vi "Lin Daten verwalten.vi"(6 "Aktionen":T6, 7 "Dateiname":string, 8 "Pfad":string, 9 "Stufen Tabelle":T5, 10 "Punkte umkehren":bool, 11 "Lin Daten":T1 {"CalGas Eingang" items=["Cal Gas 1", "Cal Gas 2", "Cal Gas 3"]; "Max Fehler (Sollwert)" format="%#_5g"; "Zeitdauer Stufe" format="%#_5g"; "Anzahl Stufen" format="%#_5g"; "Verdünnungsgas" items=["N2", "O2"]}) -> (0 "Pfad":string, 1 "Stufen Tabelle":T5, 2 "Lin Daten einzeln":T1 {"CalGas Eingang" items=["Cal Gas 1", "Cal Gas 2", "Cal Gas 3"]; "Max Fehler (Sollwert)" format="%#_5g"; "Zeitdauer Stufe" format="%#_5g"; "Anzahl Stufen" format="%#_5g"; "Verdünnungsgas" items=["N2", "O2"]}, 3 "Gefunden?":bool, 4 "Punkte umkehren":bool, 5 "Dateiname":string)   [LabVIEW 2020, in "Linearisierung v2.lvlib" / "Gasteiler.lvlib"]
uses:
  Gasteiler.lvlib
  Lin Daten verwalten Aktionen.ctl
  Lin Daten.ctl
  Visualisierungs Elemente/String - Eingabefeld.ctl
  Visualisierungs Elemente/Zahlen-Eingabefeld.ctl
  Stufen Tabelle.ctl
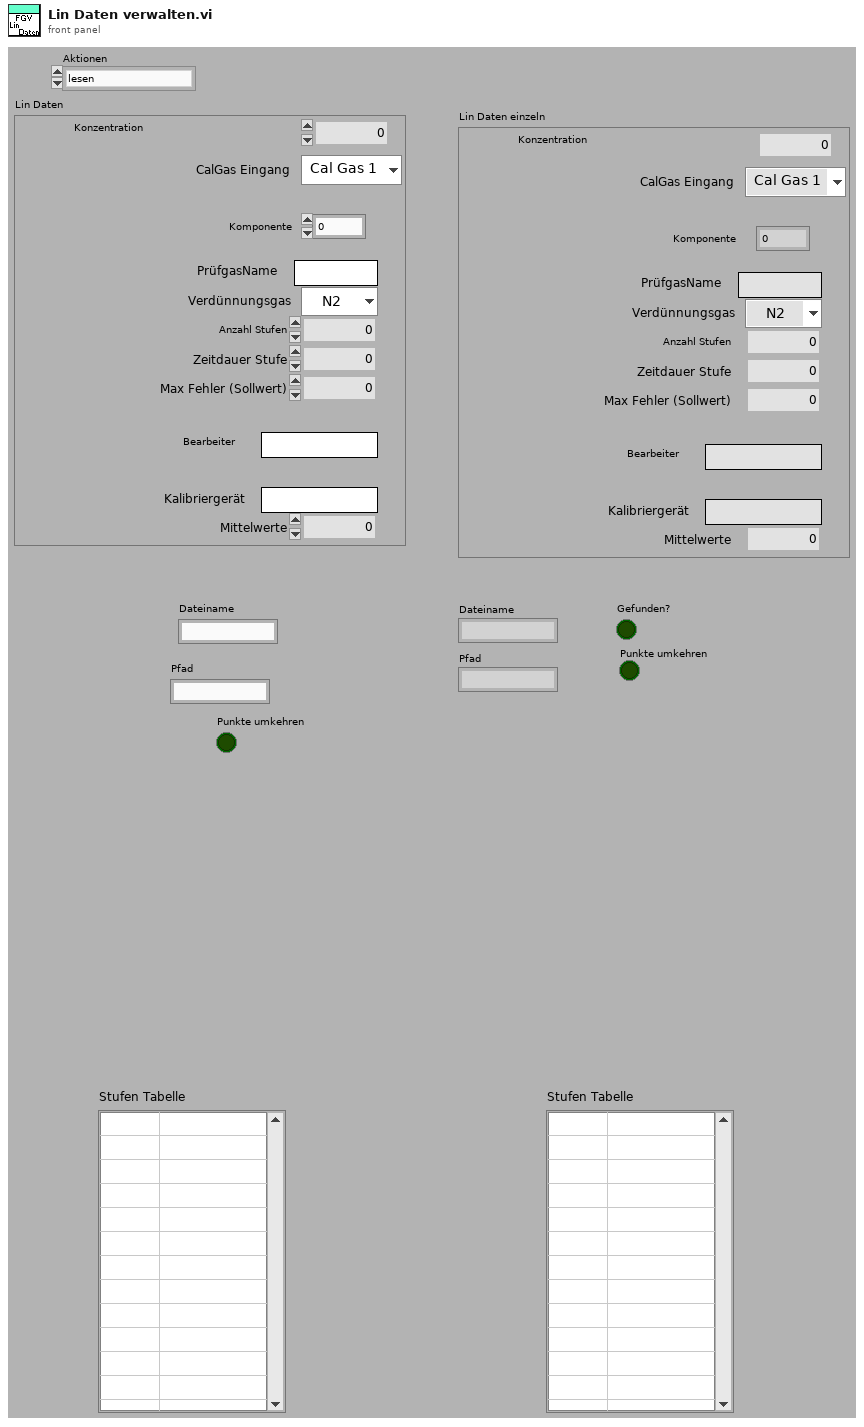
[diagram p1: front panel]
types:
  T1 = typedef "Linearisierung v2.lvlib/Gasteiler.lvlib/Lin Daten.ctl" = cluster{"PrüfgasName":T2, "Verdünnungsgas":T3, "Anzahl Stufen":T4, "Zeitdauer Stufe":T4, "Max Fehler (Sollwert)":T4, "Bearbeiter":T2, "Kalibriergerät":T2, "Mittelwerte":i32, "Komponente":u16, "CalGas Eingang":u16, "Konzentration":sgl}
  T2 = typedef "String - Eingabefeld.ctl" = string
  T3 = typedef "Linearisierung v2.lvlib/Gasteiler.lvlib/Prüfgas in.ctl" = u16
  T4 = typedef "Zahlen-Eingabefeld.ctl" = sgl
  T5 = typedef "Linearisierung v2.lvlib/Gasteiler.lvlib/Stufen Tabelle.ctl" = string[][]
  T6 = typedef "Linearisierung v2.lvlib/Gasteiler.lvlib/Lin Daten verwalten Aktionen.ctl" = enum16{"lesen", "speichern", "laden", "Lin Daten schr.", "Stufen Tabelle", "Lin Name AK", "Lin Pfad AK", "Umkehren"}
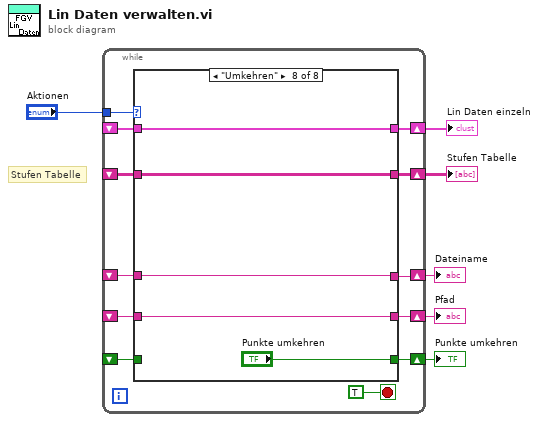
[diagram p0: block diagram]
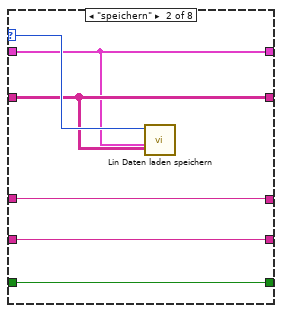
[diagram p3: hidden frame]
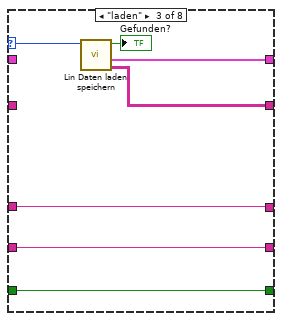
[diagram p4: hidden frame]
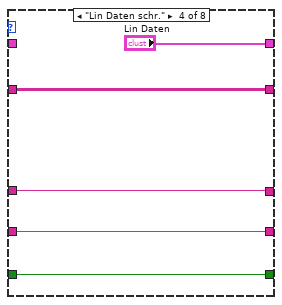
[diagram p5: hidden frame]
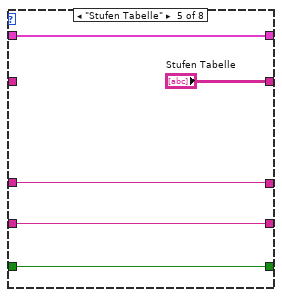
[diagram p6: hidden frame]
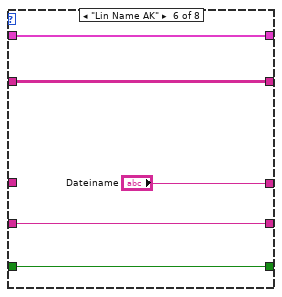
[diagram p7: hidden frame]
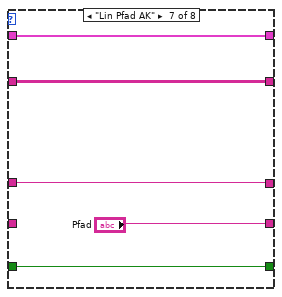
[diagram p8: hidden frame]
diagram:
  # "Stufen Tabelle"
  n1 = while {
    tunnel: "Aktionen" -> [w17]
    shift-right: [w16] -> w5
    shift-left: _ -> [w15]
    shift-right: [w13] -> w4
    shift-left: _ -> [w14]
    shift-right: [w12] -> w3
    shift-left: _ -> [w11]
    shift-right: [w10] -> w2
    shift-left: _ -> [w9]
    shift-right: [w8] -> w1
    shift-left: _ -> [w7]
    stop <- TRUE stop-if-true
    n2 = case shown="\"Umkehren\"" w17 {
      selector: w17 -> [_ w29 w36 _ _ _ _ _]
      tunnel: [w23 w27 w34 "Lin Daten" w46 w51 w54 w57] -> w16
      tunnel: w15 -> [w23 w27 _ _ w46 w51 w54 w57]
      tunnel: w14 -> [w22 w28 _ w41 _ w50 w55 w58]
      tunnel: [w22 w28 w35 w41 "Stufen Tabelle" w50 w55 w58] -> w13
      tunnel: [w21 w26 w33 w39 w44 "Dateiname" w56 w59] -> w12
      tunnel: w11 -> [w21 w26 w33 w39 w44 _ w56 w59]
      tunnel: [w20 w25 w32 w38 w43 w48 "Pfad" w60] -> w10
      tunnel: w9 -> [w20 w25 w32 w38 w43 w48 _ w60]
      tunnel: [w19 w24 w30 w37 w42 w47 w52 "Punkte umkehren"] -> w8
      tunnel: w7 -> [w19 w24 w30 w37 w42 w47 w52 _]
      frame "lesen", Default {
      }
      frame "speichern" {
        n3 = call "Lin Daten laden speichern.vi"("Stufen Tabelle"=w28, "Lin Daten"=w27, "Aktionen"=w29) -> ()  [unwired: 6 in, 3 out]
      }
      frame "laden" {
        n4 = call "Lin Daten laden speichern.vi"("Aktionen"=w36) -> ("Stufen Tabellen"=w35:T5, "Lin Daten Array"=w34:T1, "Gefunden?"=→"Gefunden?":bool)  [unwired: 8 in]
      }
      frame "Lin Daten schr." {
      }
      frame "Stufen Tabelle" {
      }
      frame "Lin Name AK" {
      }
      frame "Lin Pfad AK" {
      }
      frame "Umkehren" {
      }
    }
  }
  "Lin Daten einzeln" <- w5
  "Stufen Tabelle" <- w4
  "Dateiname" <- w3
  "Pfad" <- w2
  "Punkte umkehren" <- w1
